vi "Datalog append STATE.vi"(0 "Datalog (State) path":path, 2 "All state values":T1[](array[typedef]) {"Inertial state values"."w_z (dps)" format="%#_4f"; "Inertial state values"."a_y (g)" format="%#_4f"; "Inertial state values"."a_z (g)" format="%#_4f"; "Inertial state values"."w_y (dps)" format="%#_4f"; "Inertial state values"."a_x (g)" format="%#_4f"; "Inertial state values"."Sensor temp. (degC)" format="%#.2f"; "Inertial state values"."w_x (dps)" format="%#_4f"; "Environmental state values"."Dew point (degC)" format="%#.2f"; "Environmental state values"."Density (kg/m^3)" format="%#.3f"; "Environmental state values"."Pressure alt. (m)" format="%#.2f"; "Environmental state values"."Density alt. (m)" format="%#.2f"; "Environmental state values"."Rel. Humidity (%)" format="%#.2f"; "Environmental state values"."P_atmos (Pa)" format="%#_6f"; "Environmental state values"."Sensor temp. (degC)" format="%#.2f"; "Environmental state values"."Thermistor (degC)" format="%#.2f"}, 3 "Error in":errorcluster) -> (6 "Path out":path, 9 "Error out":errorcluster)   [LabVIEW 2015]
uses:
  Ctls/All state values (for datalog).ctl
  Ctls/Environmental state values.ctl
  Ctls/Inertial state values.ctl
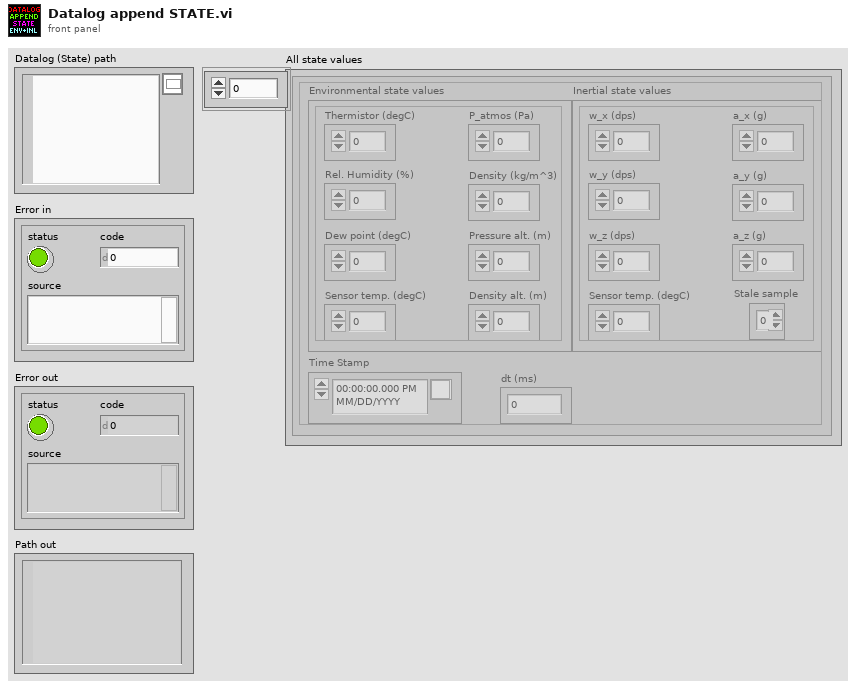
[diagram p1: front panel]
types:
  T1 = typedef "All state values (for datalog).ctl" = cluster{"Time Stamp":timestamp, "dt (ms)":i32, "Environmental state values":T2, "Inertial state values":T3}
  T2 = typedef "Environmental state values.ctl" = cluster{"Thermistor (degC)":sgl, "Sensor temp. (degC)":sgl, "P_atmos (Pa)":sgl, "Rel. Humidity (%)":sgl, "Density (kg/m^3)":sgl, "Dew point (degC)":sgl, "Pressure alt. (m)":sgl, "Density alt. (m)":sgl}
  T3 = typedef "Inertial state values.ctl" = cluster{"w_x (dps)":sgl, "w_y (dps)":sgl, "w_z (dps)":sgl, "a_x (g)":sgl, "a_y (g)":sgl, "a_z (g)":sgl, "Stale sample":u8, "Sensor temp. (degC)":sgl}
  T4 = enum16{"open", "replace", "create", "open or create", "replace or create", "replace or create with confirmation"}
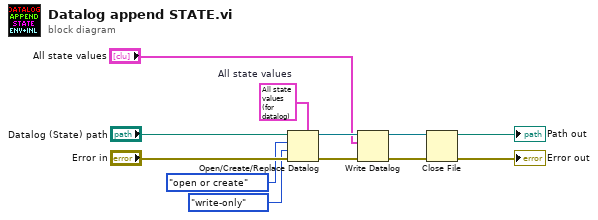
[diagram p0: block diagram]
diagram:
  w1 = T1 {"Time Stamp"=timestamp(0 s since 1904-01-01), "dt (ms)"=0, "Environmental state values"={"Thermistor (degC)"=0.0, "Sensor temp. (degC)"=0.0, "P_atmos (Pa)"=0.0, "Rel. Humidity (%)"=0.0, "Density (kg/m^3)"=0.0, "Dew point (degC)"=0.0, "Pressure alt. (m)"=0.0, "Density alt. (m)"=0.0}, "Inertial state values"={"w_x (dps)"=0.0, "w_y (dps)"=0.0, "w_z (dps)"=0.0, "a_x (g)"=0.0, "a_y (g)"=0.0, "a_z (g)"=0.0, "Stale sample"=0, "Sensor temp. (degC)"=0.0}}  # All state values
  n1 = Open/Create/Replace Datalog(5:w1, 8:"Error in", 9:enum16{"read/write", "read-only", "write-only"}."write-only" ("access (0:read/write)"), 10:T4."open or create" ("operation (0:open)"), 11:"Datalog (State) path") -> (0:w8:errorcluster, 3:w7:refnum<k1>)  [unwired: 1 in, 1 out]
  n2 = Write Datalog(4:w8, 6:"All state values", 7:w7) -> (0:w6:errorcluster, 3:w5:refnum<k1>)
  n3 = Close File(refnum=w5, error in=w6) -> (path=→"Path out":path, error out=→"Error out":errorcluster)
